vi "Receiver_Example - 2 Channel - Experiment_3.vi"() -> ()   [LabVIEW 2022 SP3]
panel:
  out "CH0":bool
  out "CH1":bool
  out "iterationsIM  2":dbl
  out "iterationsIM":dbl
  out "High-Power Image 2":T1(plugin-control)
  out "High-Power Decoded message - CH0":string
  out "High-Power BER":T2(graph)
  in  "High-Power Window Size":dbl=15.0 format="%#_6p"
  in  "Low-Power Window Size - CH0":dbl=15.0 format="%#_6p"
  out "Low-Power BER - CH0":dbl(graph)
  out "Constellation Map":cluster{"Constellation":cdb[]}[](graph)
  in  "Tab Control":enum32{"USRP Parameters", "Rx Info", "BER"}(tab)
  in  "USRP ControledParameters":T3={"Active Antenna"="RX2", "Gain (dB)"=10.0, "Carrier Frequency"=2400000000.0, "IQ Rate"=2000000.0, "Active channels"="0,1"} {"IQ Rate" format="%#_6p"; "Carrier Frequency" format="%#_6p"; "Gain (dB)" format="%#_6f"}
  in  "Device selection":refnum<k15>="RIO0"
  in  "Trigger level":dbl=0.005 format="%f"
  out "CH0":T4
  out "CH1":T4
  out "SIG valid? - CH1":bool
  out "SIG valid? - CH0":bool
  out "Frequency offset - CH1":dbl
  out "Frequency offset - CH0":dbl
  out "Coerced Parameters":T5={"IQ Rate"=100000.0, "Carrier  Freq."=100000.0, "Gain"=0.0} {"Gain" format="%#_6f"; "Carrier  Freq." format="%#_6p"; "IQ Rate" format="%#_6p"}
  out "Error out":errorcluster
  in  "Expected message LP - CH0":string="Non Critical Data\nNon Critical Data\nNon Critical Data\nNon Critical Data\nNon Critical Data"
  in  "Expected message - CH1":string="Critical Dataaaaa\nCritical Dataaaaa\nCritical Dataaaaa\nCritical Dataaaaa\nCritical Dataaaaa"
  out "Expected message LP Detected CH0":string="Non Critical Data\nNon Critical Data\nNon Critical Data\nNon Critical Data\nNon Critical Data"
  out "Expected message HP Detected CH1":string="Non Critical Data\nNon Critical Data\nNon Critical Data\nNon Critical Data\nNon Critical Data"
  in  "Boolean":bool
  in  "Boolean 3":bool
  out "Expected message HP Detected CH0":string="Non Critical Data\nNon Critical Data\nNon Critical Data\nNon Critical Data\nNon Critical Data"
  in  "Expected message HP - CH0":string="Critical Dataaaaa\nCritical Dataaaaa\nCritical Dataaaaa\nCritical Dataaaaa\nCritical Dataaaaa"
  in  "Boolean 2":bool
  out "Inst. BER HP - CH0":dbl format="%#_4g"
  out "Acc. BER HP - CH0":dbl format="%#_4g"
  out "Acum. Err HP - CH0":dbl
  out "No. Bits HP - CH0":dbl
  out "Acc. BER LP - CH0":dbl format="%#_4g"
  out "Inst. BER - CH1":dbl format="%#_4g"
  out "Inst. BER LP - CH0":dbl format="%#_4g"
  out "No. Bits - CH1":dbl
  out "No. Bits LP - CH0":dbl
  out "Acum. Err - CH1":dbl
  out "Acum. Err LP - CH0":dbl
  in  "Record BER":bool
  in  "Refresh Button":bool
  out "Acc. BER - CH1":dbl format="%#_4g"
  in  "error in (no error)":errorcluster
  out "Decoded message - CH1":string
  out "Low-Power Decoded message - CH0":string
  # "OFDM Superposition Coded Receiver"
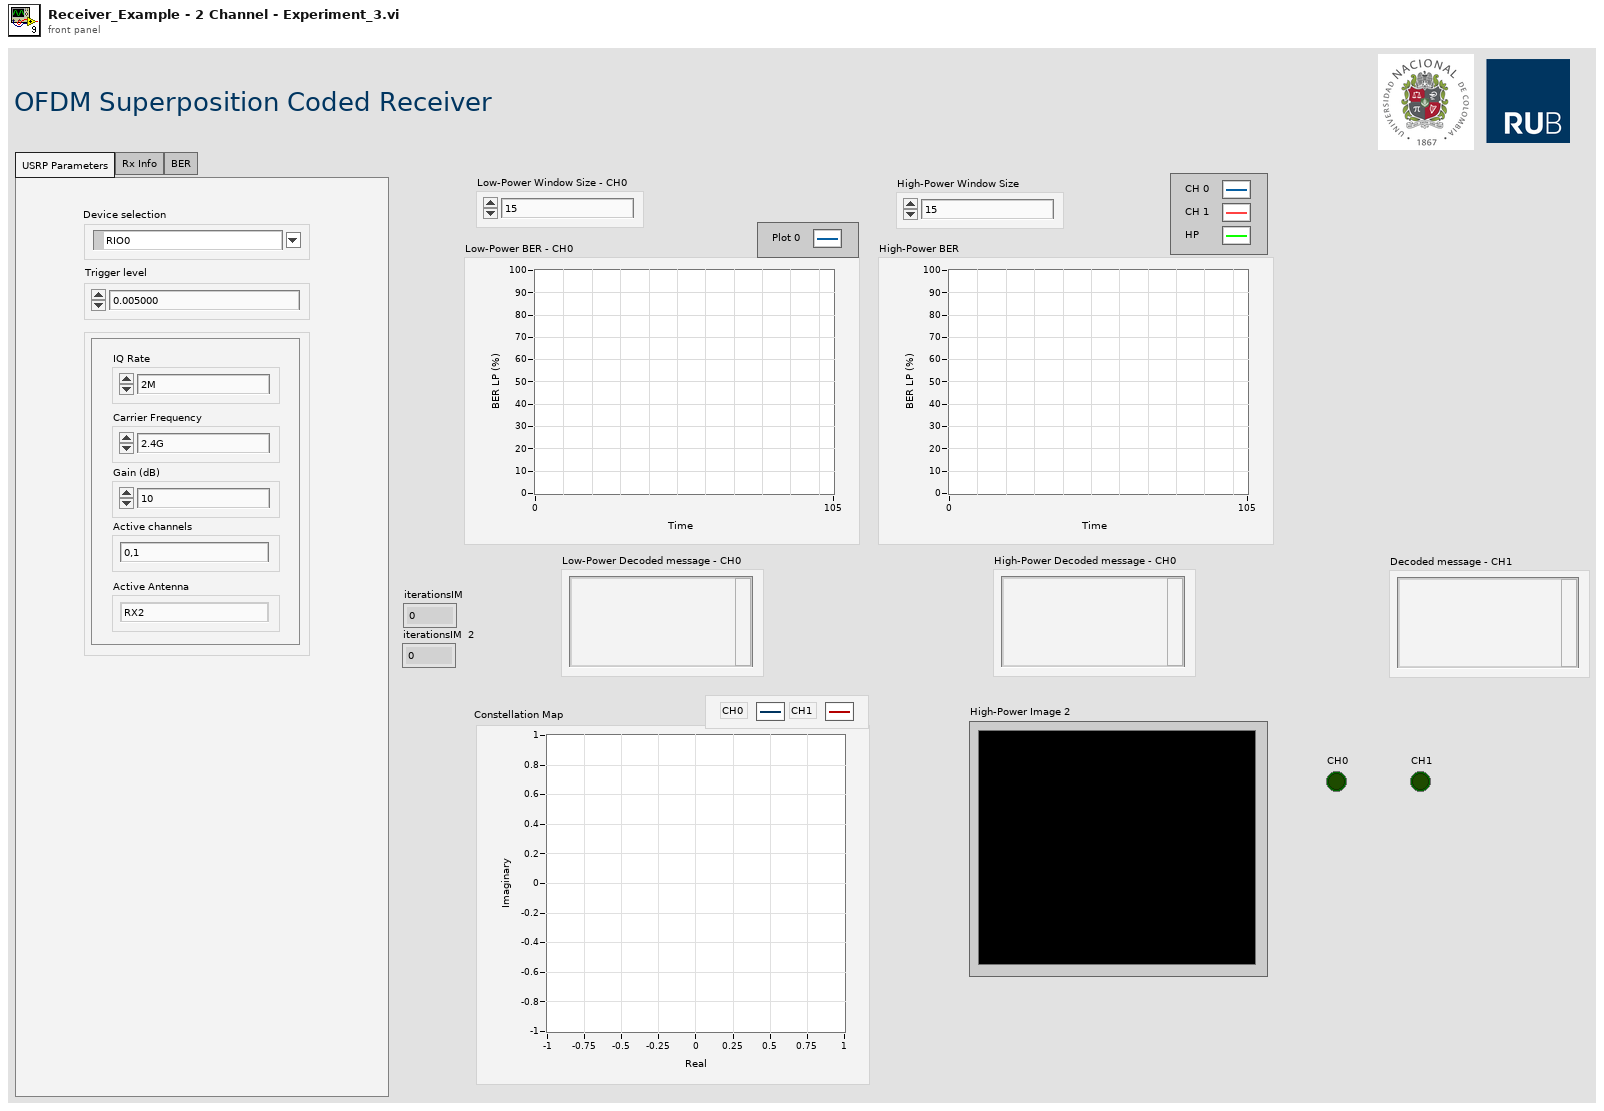
[diagram p1: front panel]
types:
  T1 = typedef "IMAQ Image.ctl" = refnum<image>
  T2 = cluster{"Graph Instantaneous BER":dbl, "Graph Instantaneous BER":dbl, "Inst. BER - CH1":dbl}
  T3 = cluster{"Active Antenna":string, "Gain (dB)":dbl, "Carrier Frequency":dbl, "IQ Rate":dbl, "Active channels":string}
  T4 = cluster{"Modulation type":enum16{"QPSK(4QAM)", "64QAM", "16QAM", "BPSK"}, "BCC rate (k/n)":enum16{"1/2", "2/3", "3/4"}}
  T5 = cluster{"IQ Rate":dbl, "Carrier  Freq.":dbl, "Gain":dbl}
  T6 = cluster{"coerced IQ rate":dbl, "coerced carrier frequency":dbl, "coerced gain":dbl}
  T7 = cluster{"Graph Instantaneous BER":dbl, "Graph Instantaneous BER":dbl, "Graph Instantaneous BER":dbl}
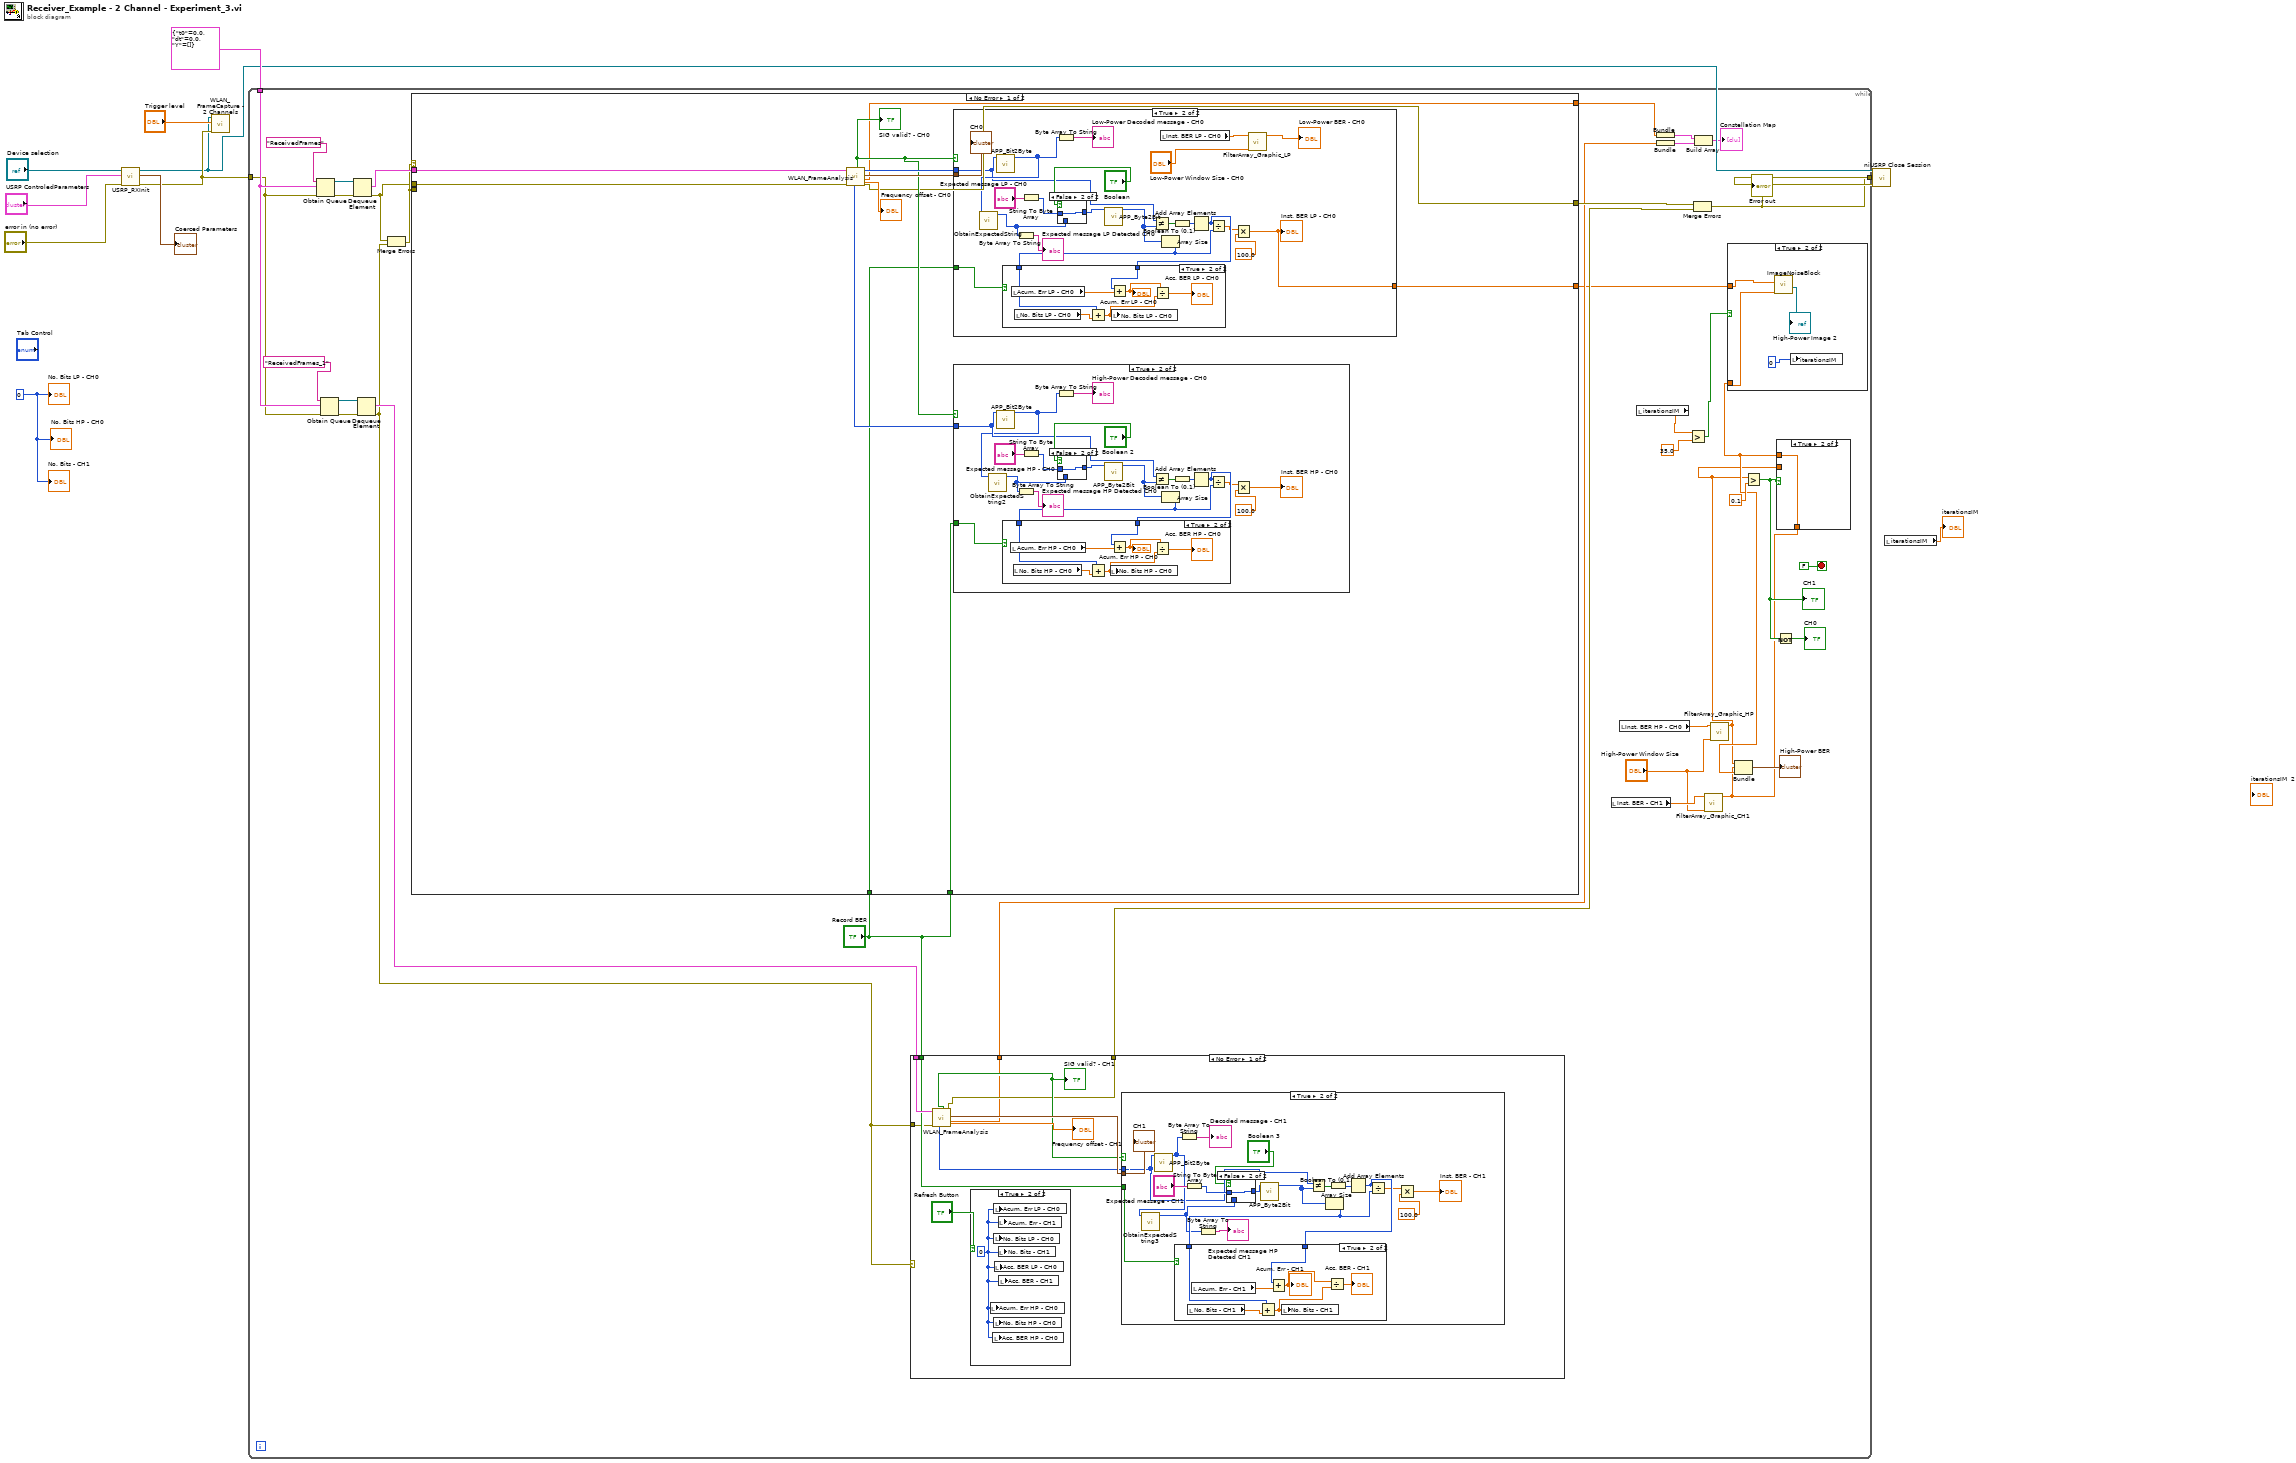
[diagram p0: block diagram]
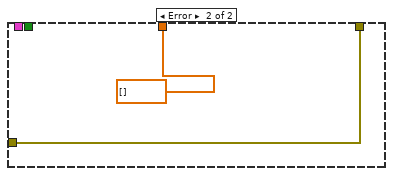
[diagram p7: hidden frame]
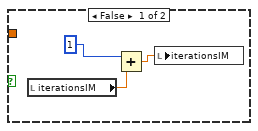
[diagram p8: hidden frame]
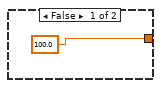
[diagram p12: hidden frame]
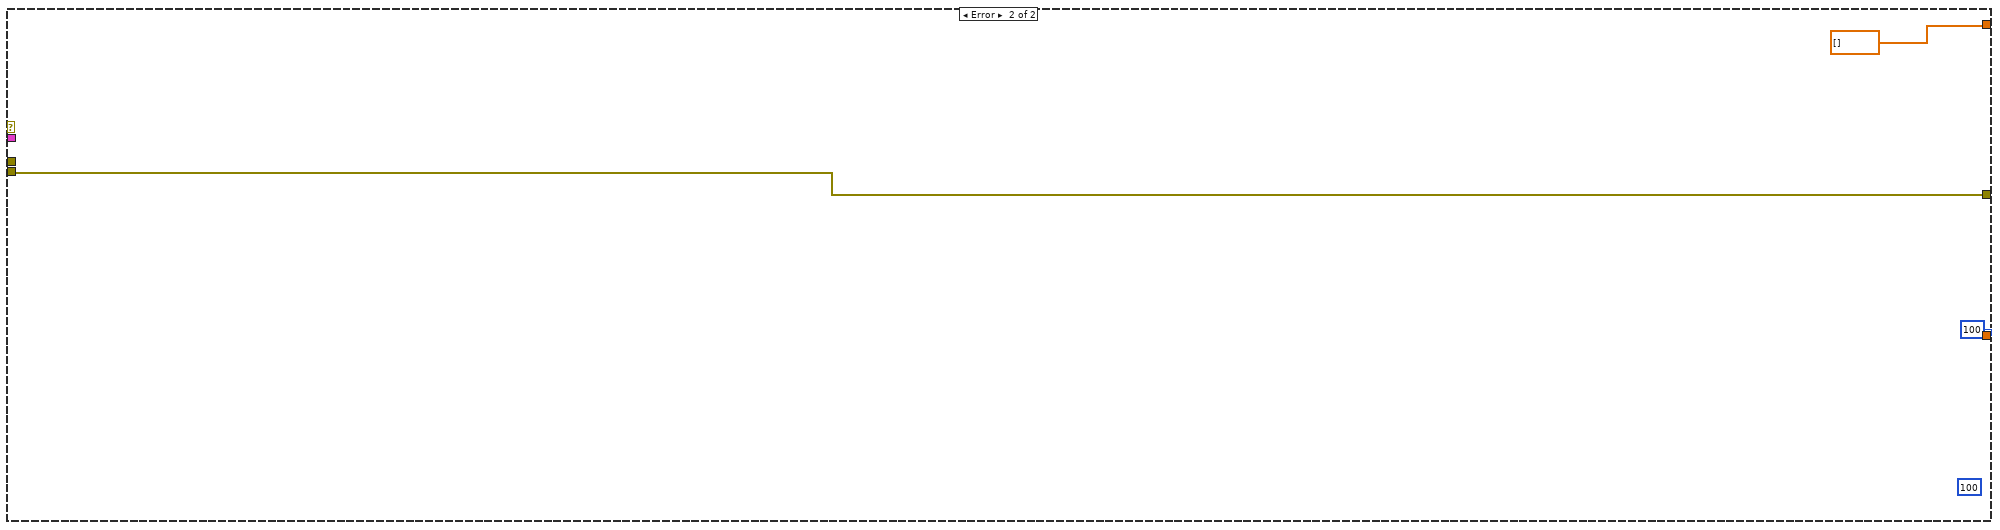
[diagram p15: hidden frame]
diagram:
  w2 = 0
  n1 = call "USRP_RXInit.vi"("device names"="Device selection", "USRP ControledParameters"="USRP ControledParameters", "error in (no error)"="error in (no error)") -> ("session handle out"=w5:refnum<k15>, "USRP CoercedParamters"=→"Coerced Parameters":T6, "error out"=w9:errorcluster)  [unwired: 5 in]
  n2 = call "WLAN_FrameCapture - 2 Channels.vi"("error in (no error)"=w9, "Trigger level"="Trigger level", "session handle"=w5) -> ()  [unwired: 8 in]
  n3 = while {
    tunnel: w9 -> [w40]
    tunnel: cluster{"t0":dbl, "dt":dbl, "Y":cdb[]} {"t0"=0.0, "dt"=0.0, "Y"=[]} ("data") -> [w41]
    tunnel: [w26] -> w6
    stop <- FALSE stop-if-true
    n4 = Obtain Queue(name (unnamed)="ReceivedFrames", element data type=w41, error in (no error)=w40) -> (queue out=w48:refnum<queue>, error out=w46:errorcluster)  [unwired: 2 in, 1 out]
    n5 = Obtain Queue(name (unnamed)="ReceivedFrames_1", element data type=w41, error in (no error)=w40) -> (queue out=w44:refnum<queue>, error out=w43:errorcluster)  [unwired: 2 in, 1 out]
    n6 = Dequeue Element(queue=w48, error in (no error)=w46) -> (element=w47:cluster{"t0":dbl, "dt":dbl, "Y":cdb[]}, error out=w37:errorcluster)  [unwired: 1 in, 2 out]
    n7 = Dequeue Element(queue=w44, error in (no error)=w43) -> (element=w29:cluster{"t0":dbl, "dt":dbl, "Y":cdb[]}, error out=w24:errorcluster)  [unwired: 1 in, 2 out]
    n8 = Merge Errors(w37, w24) -> (w38:errorcluster)
    n9 = case shown="No Error" w38 {
      tunnel: w47 -> [w107 _]
      tunnel: w38 -> [_ w171]
      tunnel: w37 -> [w104 _]
      tunnel: [w103 100] -> w19
      tunnel: [w102 dbl[] []] -> w30
      tunnel: [w101 w171] -> w28
      tunnel: "Record BER" -> [w100 _]
      tunnel: "Record BER" -> [w99 _]
      frame No Error {
        n10 = call "WLAN_FrameAnalysis.vi"("error in (no error)"=w104, "input cluster"=w107) -> ("error out"=w101:errorcluster, "Constellation"=w102:cdb[], "Modulation parameter"=w108:T4, "output bits"=w109:i8[], "Frequency offset"=→"Frequency offset - CH0":dbl, "SIG valid?"=w105:bool, "outputbitsHP"=w106:i8[])  [unwired: 3 in]
        "SIG valid? - CH0" <- w105
        n11 = case shown="True" w105 {
          tunnel: w109 -> [_ w141]
          tunnel: w108 -> [_ w159]
          tunnel: w99 -> [_ w155]
          tunnel: [100.0 w140] -> w103
          frame False {
          }
          frame True {
            n12 = call "APP_Bit2Byte.vi"("input bit stream"=w141) -> ("output byte stream"=w145:u8[])  [unwired: 10 in]
            n13 = call "ObtainExpectedString.vi"("Array"=w145) -> ("detectedMessage"=w142:i8[])  [unwired: 9 in]
            n14 = Byte Array To String(unsigned byte array=w142) -> (string=→"Expected message LP Detected CH0":string)
            n15 = String To Byte Array(string="Expected message LP - CH0") -> (unsigned byte array=w146:u8[])
            n16 = Byte Array To String(unsigned byte array=w145) -> (string=→"Low-Power Decoded message - CH0":string)
            n17 = case shown="False" "Boolean" {
              tunnel: [w161 w162] -> w148
              tunnel: w146 -> [_ w162]
              tunnel: w142 -> [w161 _]
              frame True {
              }
              frame False {
              }
            }
            n18 = call "APP_Byte2Bit.vi"("input byte stream"=w148) -> ("output bit stream"=w147:i8[])  [unwired: 10 in]
            n19 = Not Equal?(x=w141, y=w147) -> (x != y?=w157:bool[])
            n20 = local read "Inst. BER LP - CH0"() -> (w151:dbl)
            n21 = Array Size(array=w147) -> (size(s)=w154:i32)
            n22 = Boolean To (0,1)(Boolean=w157) -> (0, 1=w158:i16[])
            n23 = Add Array Elements(numeric array=w158) -> (sum=w153:i16)
            n24 = case shown="True" w155 {
              tunnel: w154 -> [_ w168]
              tunnel: w153 -> [_ w166]
              frame False {
              }
              frame True {
                n25 = local read "Acum. Err LP - CH0"() -> (w167:dbl)
                n26 = local read "No. Bits LP - CH0"() -> (w169:dbl)
                n27 = Add(x=w168, y=w169) -> (x+y=w165:dbl)
                n28 = Add(x=w166, y=w167) -> (x+y=w164:dbl)
                "Acum. Err LP - CH0" <- w164
                n29 = local write "No. Bits LP - CH0"(w165) -> ()
                n30 = Divide(x=w164, y=w165) -> (x/y=→"Acc. BER LP - CH0":dbl)
              }
            }
            n31 = Divide(x=w153, y=w154) -> (x/y=w150:dbl)
            n32 = Multiply(x=w150, y=100.0) -> (x*y=w140:dbl)
            "Inst. BER LP - CH0" <- w140
            n33 = call "FilterArray_Graphic_LP.vi"("Window Size"="Low-Power Window Size - CH0", "Instantaneous BER"=w151) -> ("Graph Instantaneous BER"=→"Low-Power BER - CH0":dbl)  [unwired: 4 in, 1 out]
            "CH0" <- w159
          }
        }
        n34 = case shown="True" w105 {
          tunnel: w106 -> [_ w114]
          tunnel: w100 -> [_ w124]
          frame False {
          }
          frame True {
            n35 = call "APP_Bit2Byte.vi"("input bit stream"=w114) -> ("output byte stream"=w113:u8[])  [unwired: 10 in]
            n36 = call "ObtainExpectedString2.vi"("Array"=w113) -> ("detectedMessage"=w112:i8[])  [unwired: 9 in]
            n37 = Byte Array To String(unsigned byte array=w112) -> (string=→"Expected message HP Detected CH0":string)
            n38 = String To Byte Array(string="Expected message HP - CH0") -> (unsigned byte array=w117:u8[])
            n39 = Byte Array To String(unsigned byte array=w113) -> (string=→"High-Power Decoded message - CH0":string)
            n40 = case shown="False" "Boolean 2" {
              tunnel: [w129 w130] -> w119
              tunnel: w117 -> [_ w130]
              tunnel: w112 -> [w129 _]
              frame True {
              }
              frame False {
              }
            }
            n41 = call "APP_Byte2Bit.vi"("input byte stream"=w119) -> ("output bit stream"=w118:i8[])  [unwired: 10 in]
            n42 = Not Equal?(x=w114, y=w118) -> (x != y?=w126:bool[])
            n43 = Array Size(array=w118) -> (size(s)=w123:i32)
            n44 = Boolean To (0,1)(Boolean=w126) -> (0, 1=w127:i16[])
            n45 = Add Array Elements(numeric array=w127) -> (sum=w122:i16)
            n46 = case shown="True" w124 {
              tunnel: w123 -> [_ w136]
              tunnel: w122 -> [_ w134]
              frame False {
              }
              frame True {
                n47 = local read "Acum. Err HP - CH0"() -> (w135:dbl)
                n48 = local read "No. Bits HP - CH0"() -> (w137:dbl)
                n49 = Add(x=w136, y=w137) -> (x+y=w133:dbl)
                n50 = local write "No. Bits HP - CH0"(w133) -> ()
                n51 = Add(x=w134, y=w135) -> (x+y=w132:dbl)
                "Acum. Err HP - CH0" <- w132
                n52 = Divide(x=w132, y=w133) -> (x/y=→"Acc. BER HP - CH0":dbl)
              }
            }
            n53 = Divide(x=w122, y=w123) -> (x/y=w121:dbl)
            n54 = Multiply(x=w121, y=100.0) -> (x*y=→"Inst. BER HP - CH0":dbl)
          }
        }
      }
      frame Error {
        (unwired) 100
      }
    }
    n55 = case shown="No Error" w24 {
      tunnel: w29 -> [w56 _]
      tunnel: "Record BER" -> [w54 _]
      tunnel: [w53 w91] -> w27
      tunnel: [w52 dbl[] []] -> w25
      tunnel: w24 -> [w51 w91]
      frame No Error {
        n56 = call "WLAN_FrameAnalysis.vi"("error in (no error)"=w51, "input cluster"=w56) -> ("error out"=w53:errorcluster, "Constellation"=w52:cdb[], "Modulation parameter"=w59:T4, "Frequency offset"=→"Frequency offset - CH1":dbl, "SIG valid?"=w55:bool, "outputbitsHP"=w57:i8[])  [unwired: 3 in, 1 out]
        "SIG valid? - CH1" <- w55
        n57 = case shown="True" "Refresh Button" {
          frame False {
          }
          frame True {
            w61 = 0
            n58 = local write "Acum. Err HP - CH0"(w61) -> ()
            n59 = local write "Acc. BER HP - CH0"(w61) -> ()
            n60 = local write "Acum. Err LP - CH0"(w61) -> ()
            n61 = local write "No. Bits LP - CH0"(w61) -> ()
            n62 = local write "No. Bits HP - CH0"(w61) -> ()
            n63 = local write "Acc. BER LP - CH0"(w61) -> ()
            n64 = local write "Acum. Err - CH1"(w61) -> ()
            n65 = local write "No. Bits - CH1"(w61) -> ()
            n66 = local write "Acc. BER - CH1"(w61) -> ()
          }
        }
        n67 = case shown="True" w55 {
          tunnel: w57 -> [_ w65]
          tunnel: w59 -> [_ w80]
          tunnel: w54 -> [_ w62]
          frame False {
          }
          frame True {
            n68 = call "APP_Bit2Byte.vi"("input bit stream"=w65) -> ("output byte stream"=w68:u8[])  [unwired: 10 in]
            n69 = call "ObtainExpectedString3.vi"("Array"=w68) -> ("detectedMessage"=w67:i8[])  [unwired: 9 in]
            n70 = Byte Array To String(unsigned byte array=w68) -> (string=→"Decoded message - CH1":string)
            n71 = String To Byte Array(string="Expected message - CH1") -> (unsigned byte array=w69:u8[])
            n72 = Byte Array To String(unsigned byte array=w67) -> (string=→"Expected message HP Detected CH1":string)
            n73 = case shown="False" "Boolean 3" {
              tunnel: [w81 w82] -> w71
              tunnel: w69 -> [_ w82]
              tunnel: w67 -> [w81 _]
              frame True {
              }
              frame False {
              }
            }
            n74 = call "APP_Byte2Bit.vi"("input byte stream"=w71) -> ("output bit stream"=w70:i8[])  [unwired: 10 in]
            n75 = Not Equal?(x=w65, y=w70) -> (x != y?=w77:bool[])
            n76 = Array Size(array=w70) -> (size(s)=w75:i32)
            n77 = Boolean To (0,1)(Boolean=w77) -> (0, 1=w78:i16[])
            n78 = Add Array Elements(numeric array=w78) -> (sum=w74:i16)
            n79 = case shown="True" w62 {
              tunnel: w75 -> [_ w88]
              tunnel: w74 -> [_ w86]
              frame False {
              }
              frame True {
                n80 = local read "No. Bits - CH1"() -> (w89:dbl)
                n81 = local read "Acum. Err - CH1"() -> (w87:dbl)
                n82 = Add(x=w88, y=w89) -> (x+y=w85:dbl)
                n83 = Add(x=w86, y=w87) -> (x+y=w84:dbl)
                "Acum. Err - CH1" <- w84
                n84 = local write "No. Bits - CH1"(w85) -> ()
                n85 = Divide(x=w84, y=w85) -> (x/y=→"Acc. BER - CH1":dbl)
              }
            }
            n86 = Divide(x=w74, y=w75) -> (x/y=w72:dbl)
            n87 = Multiply(x=w72, y=100.0) -> (x*y=→"Inst. BER - CH1":dbl)
            "CH1" <- w80
          }
        }
      }
      frame Error {
      }
    }
    n88 = local read "Inst. BER - CH1"() -> (w17:dbl)
    n89 = local read "Inst. BER HP - CH0"() -> (w18:dbl)
    n90 = local read "iterationsIM"() -> (w36:dbl)
    n91 = Bundle("Constellation"=w30) -> (w33:cluster{"Constellation":cdb[]})  [unwired: 1 in]
    n92 = Bundle("Constellation"=w25) -> (w32:cluster{"Constellation":cdb[]})  [unwired: 1 in]
    n93 = Greater?(x=w36, y=35.0) -> (0:w35:bool)
    n94 = Merge Errors(w28, w27) -> (w26:errorcluster)
    "Error out" <- w26
    n95 = Build Array(w33, w32) -> (→"Constellation Map":cluster{"Constellation":cdb[]}[])
    n96 = call "FilterArray_Graphic_CH1.vi"("Window Size"="High-Power Window Size", "Instantaneous BER"=w17) -> ("Graph Instantaneous BER"=w12:dbl)  [unwired: 4 in, 1 out]
    n97 = call "FilterArray_Graphic_HP.vi"("Window Size"="High-Power Window Size", "Instantaneous BER"=w18) -> ("Graph Instantaneous BER"=w13:dbl)  [unwired: 4 in, 1 out]
    n98 = Greater?(x=w13, y=0.1) -> (0:w20:bool)
    "CH1" <- w20
    n99 = case shown="True" w20 {
      tunnel: [w49 w50] -> w14
      tunnel: w12 -> [_ w50]
      tunnel: w13 -> [w49 _]
      frame False {
      }
      frame True {
      }
    }
    n100 = case shown="True" w35 {
      tunnel: w14 -> [_ w98]
      tunnel: w19 -> [_ w95]
      frame False {
        n101 = local read "iterationsIM"() -> (w94:dbl)
        n102 = Add(x=1, y=w94) -> (x+y=w93:dbl)
        n103 = local write "iterationsIM"(w93) -> ()
      }
      frame True {
        n104 = call "ImageNoiseBlock.vi"("BERLP"=w95, "BERHP"=w98) -> ("High-Power Image"=→"High-Power Image 2":T1)  [unwired: 8 in]
        n105 = local write "iterationsIM"(0) -> ()
      }
    }
    n106 = Bundle("Graph Instantaneous BER"=w13, "Graph Instantaneous BER"=w12, "Graph Instantaneous BER"=w14) -> (→"High-Power BER":T7)  [unwired: 1 in]
    n107 = Not(x=w20) -> (.not. x?=→"CH0":bool)
  }
  n108 = call <instrlib>:"niUSRP Close Session.vi"("session handle"=w5, "error in (no error)"=w6) -> ()  [unwired: 13 in, 1 out]
  n109 = local read "iterationsIM"() -> (→"iterationsIM":dbl)
  "No. Bits LP - CH0" <- w2
  "No. Bits - CH1" <- w2
  "No. Bits HP - CH0" <- w2
